vi "Read IMU.vi"(8 "error in (no error)":errorcluster) -> (0 "error out":errorcluster, 3 "Output Angle":dbl format="%#_13g")   [LabVIEW 2015]
uses:
  <vilib>/myRIO/Instrument Drivers/Onboard IO/I2C/typedefs/I2C User Configuration.ctl
  <vilib>/myRIO/Instrument Drivers/Onboard IO/I2C/typedefs/I2C Transfer Rate.ctl
  <vilib>/myRIO/Instrument Drivers/Onboard IO/I2C/typedefs/I2C Reference.ctl
  <vilib>/myRIO/Common/Instrument Driver Framework/Utilities/typedefs/myRIO Generic Hardware Reference.ctl
  <vilib>/myRIO/Common/Instrument Driver Framework/Utilities/typedefs/Hardware Version Enum.ctl
  <vilib>/myRIO/Common/Instrument Driver Framework/Utilities/typedefs/myRIO v1.0 Reference.ctl
  <vilib>/myRIO/Common/Instrument Driver Framework/Utilities/typedefs/Generic FPGA Reference.ctl
  <vilib>/myRIO/Common/Instrument Driver Framework/myRIO v1.0/I2C/typedefs/I2C Channels Enum.ctl
  <vilib>/myRIO/Instrument Drivers/Onboard IO/I2C/typedefs/I2C Configuration.ctl
  <vilib>/userdefined/High Color/nirio_resource_hc.ctl
  <vilib>/myRIO/Common/Instrument Driver Framework/Utilities/vis/Is FPGA Ref Available.vi
  <vilib>/myRIO/Common/Instrument Driver Framework/myRIO v1.0/I2C/vis/myRIO v1.1 Open I2C.vi
  <vilib>/myRIO/Instrument Drivers/Onboard IO/I2C/vis/Configure.vi
  <vilib>/myRIO/Instrument Drivers/Onboard IO/I2C/vis/Write.vi
  <vilib>/myRIO/Instrument Drivers/Onboard IO/I2C/vis/Read.vi
  <vilib>/myRIO/Common/Instrument Driver Framework/Utilities/vis/Validate Channels.vi
  <vilib>/myRIO/Common/Instrument Driver Framework/myRIO v1.0/I2C/vis/myRIO v1.0 Reserve I2C.vi
  <vilib>/myRIO/Common/Instrument Driver Framework/myRIO v1.0/I2C/vis/myRIO v1.0 Build MUX Configuration I2C.vi
  <vilib>/myRIO/Common/Instrument Driver Framework/myRIO v1.0/Resource Manager/vis/myRIO v1.0 Reserve Channel List.vi
  <vilib>/myRIO/Common/Instrument Driver Framework/myRIO v1.0/Resource Manager/vis/myRIO v1.0 Create Configuration List.vi
  <vilib>/myRIO/Common/Instrument Driver Framework/myRIO v1.0/Resource Manager/vis/myRIO v1.0 Reserve Channel.vi
  <vilib>/myRIO/Common/Instrument Driver Framework/myRIO v1.0/Resource Manager/vis/myRIO v1.0 Unreserve Channel.vi
  <vilib>/myRIO/Common/Instrument Driver Framework/myRIO v1.0/Resource Manager/vis/myRIO v1.0 Build Mutex Name.vi
  <vilib>/Utility/VariantDataType/GetNumericInfo.vi
  <vilib>/Utility/error.llb/Error Cluster From Error Code.vi
  <vilib>/myRIO/Common/Instrument Driver Framework/myRIO v1.0/myRIO v1.1 Open.vi
  <vilib>/myRIO/Common/Instrument Driver Framework/Utilities/vis/IO Manager.vi
  <vilib>/myRIO/Common/Instrument Driver Framework/Utilities/vis/Configuration Manager.vi
  <vilib>/myRIO/Common/Instrument Driver Framework/myRIO v1.0/Resource Manager/vis/myRIO v1.0 Configure IO.vi
  <vilib>/myRIO/Common/Instrument Driver Framework/myRIO v1.0/myRIO v1.0 Close.vi
  <vilib>/myRIO/Common/Instrument Driver Framework/myRIO v1.0/I2C/vis/myRIO v1.0 Configure I2C.vi
  <vilib>/myRIO/Common/Instrument Driver Framework/myRIO v1.0/I2C/vis/myRIO v1.0 Write I2C.vi
  <vilib>/myRIO/Common/Instrument Driver Framework/myRIO v1.0/I2C/vis/myRIO v1.0 Read I2C.vi
  <vilib>/myRIO/Express VI/Onboard IO/I2C/I2C Express VI.xnode
  <vilib>/myRIO/Instrument Drivers/Onboard IO/I2C/vis/myRIO I2C Open.xnode
  <vilib>/myRIO/Instrument Drivers/Onboard IO/I2C/I2C.lvlib
panel:
  out "MSB":u8[](array[numeric]) format="%b"
  out "LSB":u8[](array[numeric]) format="%b"
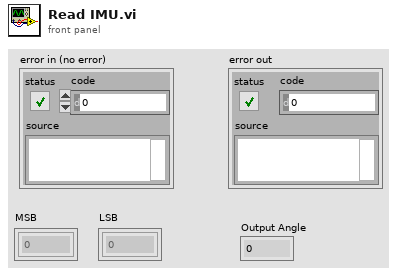
[diagram p1: front panel]
types:
  T1 = typedef "I2C.lvlib/I2C Reference.ctl" = cluster{"myRIO Reference":T2, "I2C Channels Enum":T6, "I2C Configuration":T7}
  T2 = typedef "myRIO Generic Hardware Reference.ctl" = cluster{"myRIO Model":T3, "myRIO Hardware Reference":T4}
  T3 = typedef "Hardware Version Enum.ctl" = enum16{"Unknown", "myRIO-1900", "myRIO-1950", "roboRIO"}
  T4 = typedef "myRIO v1.0 Reference.ctl" = cluster{"Generic FPGA Reference":T5, "Allow multiple opens":bool}
  T5 = typedef "Generic FPGA Reference.ctl" = refnum<k20>
  T6 = typedef "I2C Channels Enum.ctl" = enum16{"Not Connected", "A/I2C", "B/I2C", "I2C/I2C"}
  T7 = typedef "I2C.lvlib/I2C Configuration.ctl" = cluster{"I2C Transfer Rate":T8}
  T8 = typedef "I2C.lvlib/I2C Transfer Rate.ctl" = enum16{"Standard mode (100 kbps)", "Fast mode (400 kbps)"}
  T9 = typedef "I2C.lvlib/I2C User Configuration.ctl" = cluster{"I2C Transfer Rate":T8}
  T10 = typedef "nirio_resource_hc.ctl" = tag
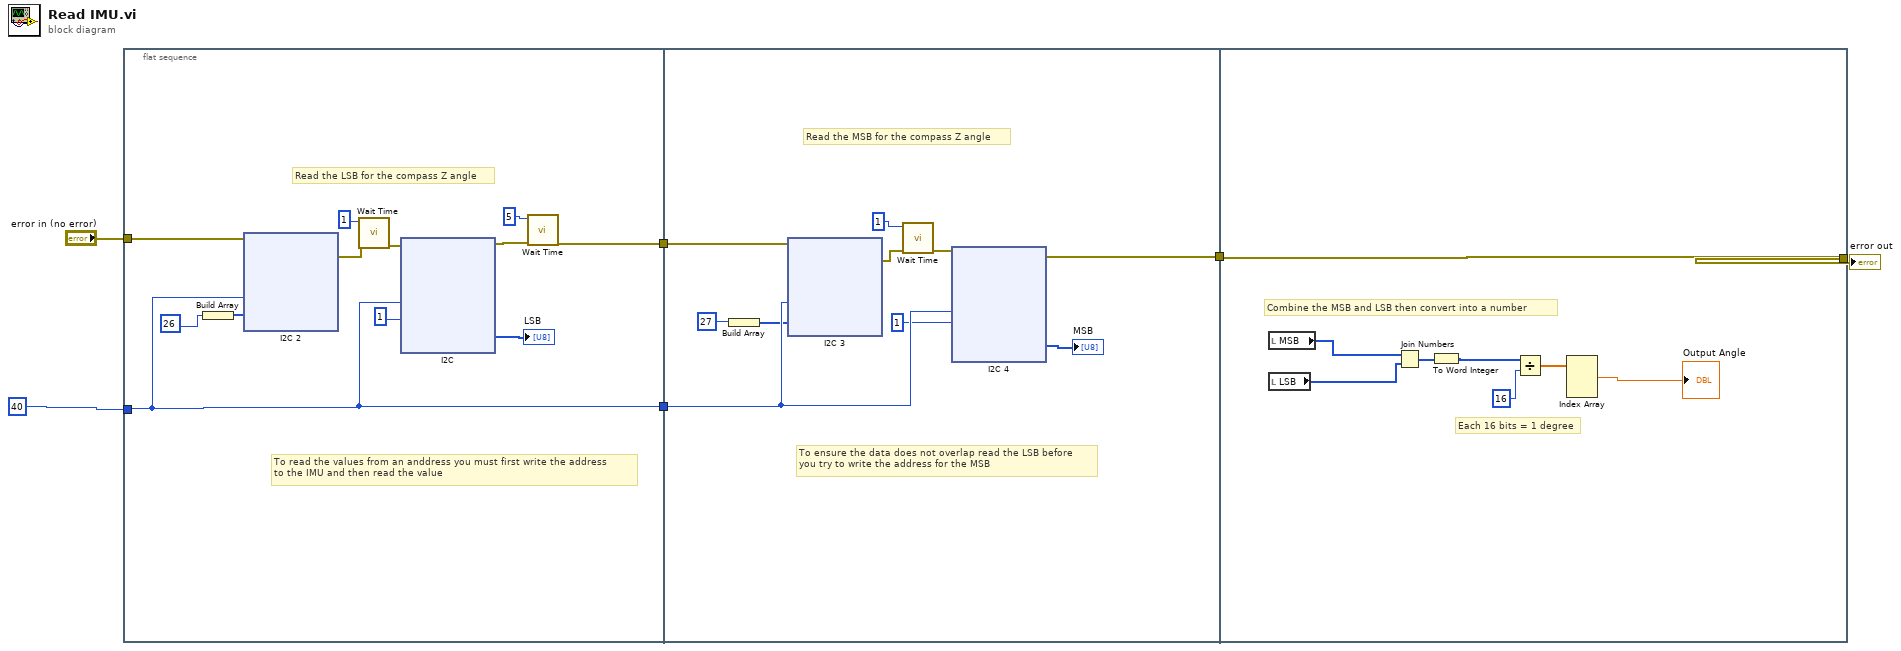
[diagram p0: block diagram]
diagram:
  n1 = flat-sequence {
    tunnel: [w10] -> w5
    tunnel: [w9] -> w4
    tunnel: 40 -> [w9]
    tunnel: "error in (no error)" -> [w7]
    tunnel: w5 -> [w105]
    tunnel: [w104] -> w3
    tunnel: w4 -> [w103]
    tunnel: w3 -> [w190]
    tunnel: [w190] -> w2
    frame #0 {
      # "To read the values from an anddress you must first write the address \nto the IMU and then read the value"
      # "Read the LSB for the compass Z angle"
      n2 = Build Array(26) -> (w16:i32[])
      n3 = xnode "I2C 2"("Slave Address (7-bit)"=w9, "Bytes to Write"=w16, "error in (no error)"=w7) -> ("error out"=w14:errorcluster)
      n4 = call "Wait Time.vi"("error in (no error)"=w14, "Wait Time (ms)"=1) -> ("error out"=w13:errorcluster)  [unwired: 9 in]
      n5 = xnode "I2C"("Slave Address (7-bit)"=w9, "Byte Count"=1, "error in (no error)"=w13) -> ("Bytes Read"=→"LSB":u8[], "error out"=w11:errorcluster)
      n6 = call "Wait Time.vi"("error in (no error)"=w11, "Wait Time (ms)"=5) -> ("error out"=w10:errorcluster)  [unwired: 9 in]
    }
    frame #1 {
      # "To ensure the data does not overlap read the LSB before \nyou try to write the address for the MSB"
      # "Read the MSB for the compass Z angle"
      n7 = Build Array(27) -> (w99:i32[])
      n8 = xnode "I2C 3"("Slave Address (7-bit)"=w103, "Bytes to Write"=w99, "error in (no error)"=w105) -> ("error out"=w97:errorcluster)
      n9 = call "Wait Time.vi"("error in (no error)"=w97, "Wait Time (ms)"=1) -> ("error out"=w96:errorcluster)  [unwired: 9 in]
      n10 = xnode "I2C 4"("Slave Address (7-bit)"=w103, "Byte Count"=1, "error in (no error)"=w96) -> ("Bytes Read"=→"MSB":u8[], "error out"=w104:errorcluster)
    }
    frame #2 {
      # "Each 16 bits = 1 degree"
      # "Combine the MSB and LSB then convert into a number"
      n11 = local read "MSB"() -> (w184:u8[])
      n12 = local read "LSB"() -> (w185:u8[])
      n13 = Join Numbers(hi=w184, lo=w185) -> ((hi.lo)=w189:u16[])
      n14 = To Word Integer(number=w189) -> (16bit integer=w183:i16[])
      n15 = Divide(x=w183, y=16) -> (x/y=w188:dbl[])
      n16 = Index Array(array=w188) -> (element #1=→"Output Angle":dbl)  [unwired: 3 in, 2 out]
    }
  }
  "error out" <- w2
